vi "autobroadsidev4.vi"() -> ()   [LabVIEW 2012, in "MainProject.lvrbt"]
uses:
  MainProject.lvrbt
  <vilib>/NXT/Dual Mode Library/Waits/Wait_Num(msec).vi
  <vilib>/NXT/Hardware/Plugins/Tetrix DC Motor/TetrixDCMotorAddress.ctl
  <vilib>/NXT/LegoClasses/BrickReference/BrickReference.lvclass
  <vilib>/NXT/Subs/LVHSConnector.ctl
  <vilib>/NXT/NXTIO Xnodes/NXTIONodeSubVIs/TETRIX IO Check Battery.vi
  <vilib>/NXT/NXTIO Xnodes/NXTIOXNode/NXTIO.xnode
  <vilib>/NXT/NXTIO Xnodes/AddressXNode/NXTIOAddress.xnode
  <vilib>/NXT/NXTIO Xnodes/NXTIONodeSubVIs/TETRIX IO Stop DC Motors.vi
  Drivers/AutoControl3.ctl
  <vilib>/NXT/Block Support/NXT_InputPort.ctl
  <vilib>/NXT/HiTechnic/HiTechnic Controls/HiTechnic Port.ctl
  Drivers/AutoDriverControl.ctl
  FTC 2012 - 2013/Controls/SpeedControl.ctl
  <vilib>/NXT/Dual Mode Library/Sound/Tone.vi
  <vilib>/NXT/Dual Mode Library/Waits/Wait_Num.vi
  <vilib>/NXT/Hardware/Plugins/Tetrix 180 deg Servo/Tetrix180ServoAddress.ctl
  <vilib>/NXT/NXTIO Xnodes/NXTIONodeSubVIs/TETRIX IO Move Servos.vi
  Drivers/LineCountColorCtl.ctl
panel:
  out "Line Color":string="Black"
  in  "Dramatic Mode":bool
  out "Color":string="Black"
  out "Sector (0-9)":i16
  out "Enabled":bool
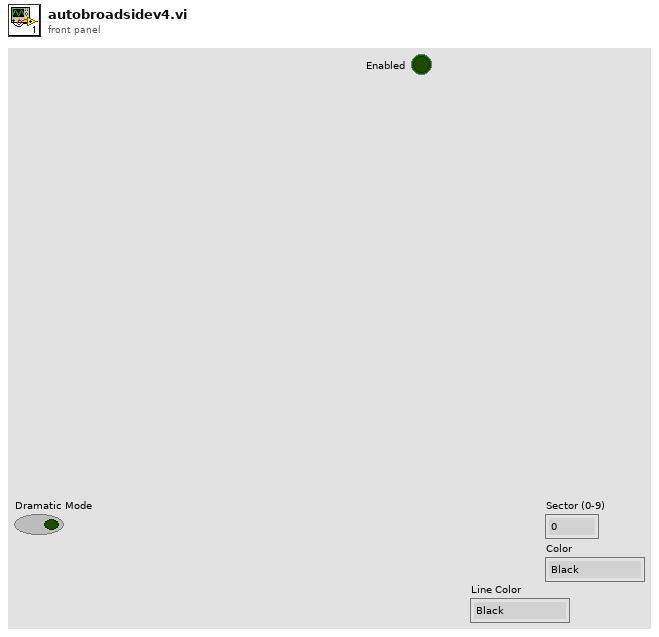
[diagram p1: front panel]
types:
  T1 = typedef "HiTechnic Port.ctl" = cluster{"Port":T2, "MUX Port":u8}
  T2 = typedef "NXT_InputPort.ctl" = u8
  T3 = typedef "TetrixDCMotorAddress.ctl" = i16
  T4 = typedef "LVHSConnector.ctl" = refnum<class "BrickReference.lvclass">
  T5 = typedef "Tetrix180ServoAddress.ctl" = i16
  T6 = typedef "AutoDriverControl.ctl" = enum16{"Init", "Forward", "Reverse", "Left", "Right", "Brake"}
  T7 = typedef "AutoControl3.ctl" = enum16{"FindIRBasket", "DropBLK", "DrvToEndOfBaskets", "DrvAroundBaskets", "AlignWithRamp", "ParkOnRamp", "Stop"}
  T8 = cluster{"Tetrix180Servo":T5, "Tetrix180Servo 2":T5, "Tetrix180Servo 3":T5, "Tetrix180Servo 4":T5}
  T9 = typedef "LineCountColorCtl.ctl" = enum16{"Init/Reset", "Check"}
  T10 = typedef "SpeedControl.ctl" = enum16{"Fast", "Medium", "Slow"}
  T11 = cluster{"Tetrix180Servo":T5, "Tetrix180Servo":T5, "Tetrix180Servo":T5, "Tetrix180Servo":T5}
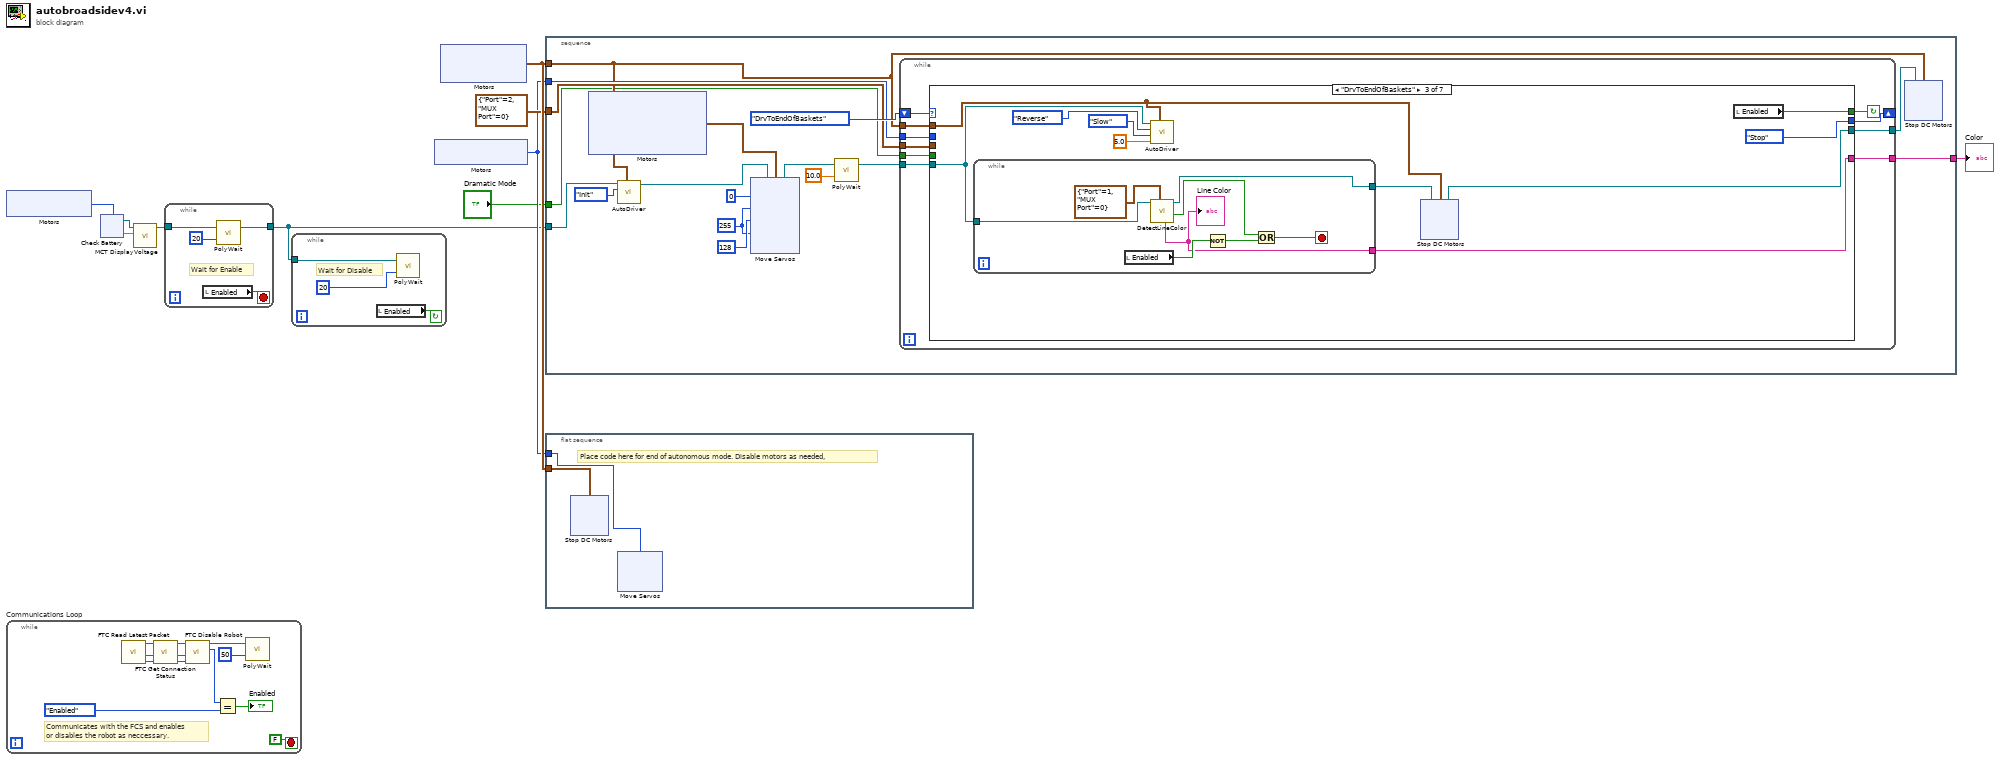
[diagram p0: block diagram]
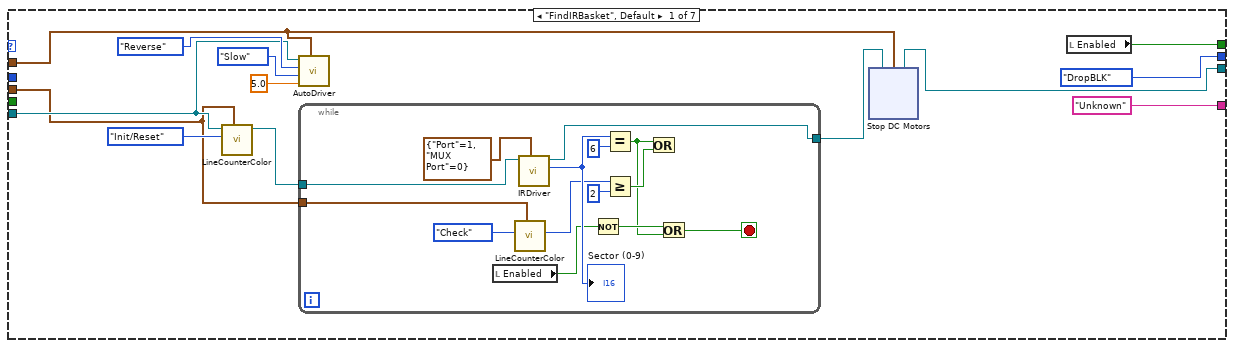
[diagram p2: hidden frame]
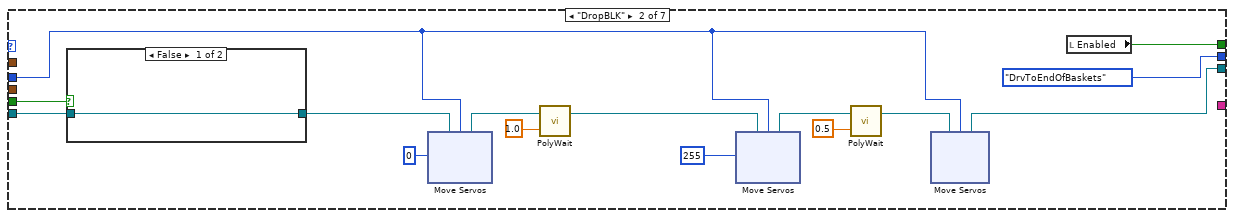
[diagram p3: hidden frame]
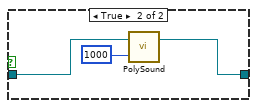
[diagram p4: hidden frame]
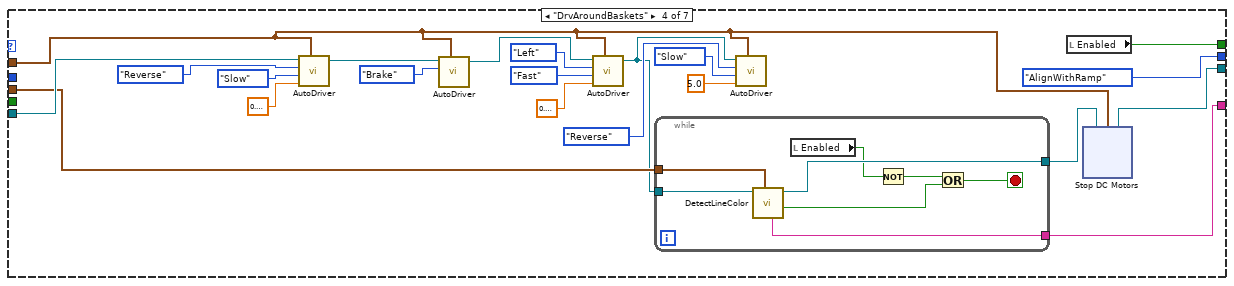
[diagram p5: hidden frame]
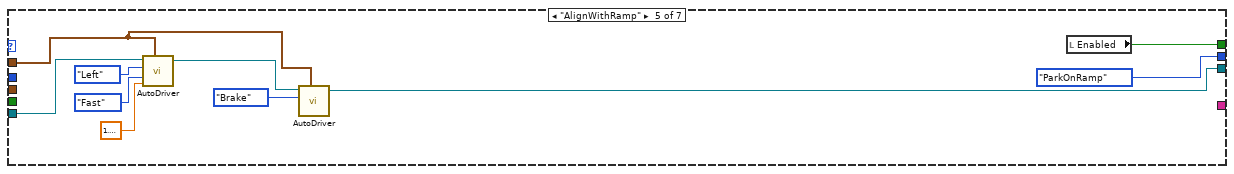
[diagram p6: hidden frame]
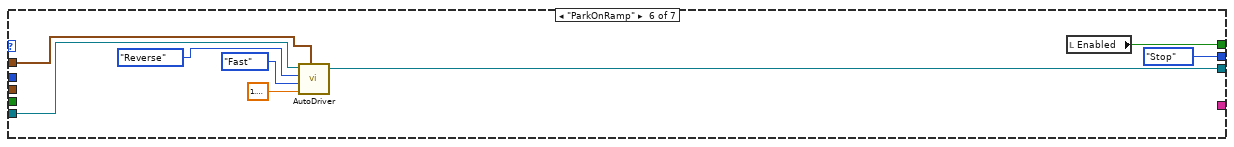
[diagram p7: hidden frame]
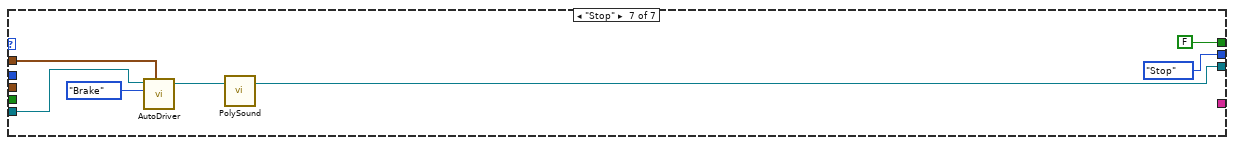
[diagram p8: hidden frame]
diagram:
  n1 = xnode "Motors"() -> ("Motor"=w5:T3)
  n2 = while "Communications Loop" {
    stop <- FALSE stop-if-true
    # "Communicates with the FCS and enables \nor disables the robot as neccessary."
    n3 = call <vilib>:"FTC Read Latest Packet.vi"() -> ("Packet Received?"=w20:bool, "Stopped?"=w19:bool, "NXT"=w22:T4)  [unwired: 6 in, 3 out]
    n4 = call <vilib>:"FTC Get Connection Status.vi"("Packet Received?"=w20, "Stopped?"=w19, "NXT"=w22) -> ("Online?"=w12:bool, "Stopped?"=w13:bool, "NXT"=w21:T4)  [unwired: 5 in]
    n5 = call <vilib>:"FTC Disable Robot.vi"("Online?"=w12, "Stopped?"=w13, "NXT"=w21) -> ("Enabled?"=w15:enum16{"Disabled", "Enabled"}, "NXT"=w17:T4)  [unwired: 3 in]
    n6 = Equal?(x=w15, y=enum16{"Disabled", "Enabled"}."Enabled") -> (x = y?=→"Enabled":bool)
    n7 = call-poly <vilib>:"PolyWait.vi"("Time (100 msec)"=u32 50 ("Time (msec)"), "NXT"=w17) -> ()  [unwired: 2 in, 1 out]
  }
  n8 = xnode "Check Battery"("Motors"=w5) -> ("Voltage 1"=w9:sgl, "NXT"=w10:T4)  [unwired: 1 in]
  n9 = call <vilib>:"MCT DisplayVoltage.vi"("Motor Voltage"=w9, "NXT"=w10) -> ("NXT"=w8:T4)  [unwired: 9 in]
  n10 = while {
    tunnel: [w25] -> w2
    tunnel: w8 -> [w23]
    stop <- w24 stop-if-true
    # "Wait for Enable"
    n11 = local read "Enabled"() -> (w24:bool)
    n12 = call-poly <vilib>:"PolyWait.vi"("Time (100 msec)"=u32 20 ("Time (msec)"), "NXT"=w23) -> ("NXT"=w25:T4)  [unwired: 2 in]
  }
  n13 = while {
    tunnel: w2 -> [w27]
    stop <- w29 continue-if-true
    # "Wait for Disable"
    n14 = local read "Enabled"() -> (w29:bool)
    n15 = call-poly <vilib>:"PolyWait.vi"("Time (100 msec)"=u32 20 ("Time (msec)"), "NXT"=w27) -> ()  [unwired: 2 in, 1 out]
  }
  n16 = xnode "Motors"() -> ("Motor"=w4:T5)
  n17 = xnode "Motors"() -> ("Motor"=w7:cluster{"TetrixDCMotor":T3, "TetrixDCMotor":T3})
  n18 = stacked-sequence {
    tunnel: w7 -> [w39]
    tunnel: w2 -> [w44]
    tunnel: T1 {"Port"=2, "MUX Port"=0} ("Port/MUX") -> [w45]
    tunnel: w4 -> [w41]
    tunnel: [w40] -> w3
    tunnel: "Dramatic Mode" -> [w30]
    frame #0 {
      w33 = u8 255 ("Position 2")
      n19 = xnode "Motors"() -> ("Motor"=w36:T11)
      n20 = call "AutoDriver.vi"("NXT In"=w44, "Motors"=w39, "Direction"=AutoDriverControl."Init") -> ("NXT Out"=w43:T4)  [unwired: 5 in]
      n21 = xnode "Move Servos"("Position 4"=w33, "Position 3"=u8 128 ("Position 5"), "Position 2"=w33, "Position 1"=u8 0, "Servos"=w36, "NXT"=w43) -> ("NXT"=w37:T4)
      n22 = call-poly <vilib>:"PolyWait.vi"("Time (1 sec)"=sgl 10.0, "NXT"=w37) -> ("NXT"=w32:T4)  [unwired: 2 in]
      n23 = while {
        tunnel: w39 -> [w78]
        tunnel: w32 -> [w77]
        shift-right: [w76] -> _
        shift-left: AutoControl3."DrvToEndOfBaskets" -> [w75]
        tunnel: w45 -> [w74]
        tunnel: w41 -> [w72]
        tunnel: [w71] -> w40
        tunnel: [w70] -> w38
        tunnel: w30 -> [w69]
        stop <- w73 continue-if-true
        n24 = case shown="\"DrvToEndOfBaskets\"" w75 {
          tunnel: w78 -> [w86 _ w154 w178 w215 w230 w238]
          tunnel: w77 -> [w87 w120 w155 w198 w214 w231 w237]
          tunnel: [AutoControl3."DropBLK" AutoControl3."DrvToEndOfBaskets" AutoControl3."Stop" AutoControl3."AlignWithRamp" AutoControl3."ParkOnRamp" AutoControl3."Stop" AutoControl3."Stop"] -> w76
          tunnel: w74 -> [w79 _ _ w191 _ _ _]
          tunnel: [w83 w119 w161 w185 w217 w225 FALSE] -> w73
          tunnel: w72 -> [_ w114 _ _ _ _ _]
          tunnel: ["Unknown" ("Color") _ w153 w186 _ _ _] -> w71
          tunnel: [w82 w118 w156 w179 w216 w224 w232] -> w70
          tunnel: w69 -> [_ w113 _ _ _ _ _]
          frame "FindIRBasket", Default {
            n25 = call "LineCounterColor.vi"("Port/MUX"=w79, "Enum"=LineCountColorCtl."Init/Reset", "NXT In"=w87) -> ("NXT Out"=w81:T4)  [unwired: 7 in, 1 out]
            n26 = call "AutoDriver.vi"("NXT In"=w87, "Motors"=w86, "Direction"=AutoDriverControl."Reverse", "Speed"=SpeedControl."Slow", "Time (1 sec)"=sgl 5.0) -> ()  [unwired: 3 in, 1 out]
            n27 = while {
              tunnel: w81 -> [w109]
              tunnel: w79 -> [w105]
              tunnel: [w106] -> w84
              stop <- w102 stop-if-true
              n28 = local read "Enabled"() -> (w103:bool)
              n29 = call "LineCounterColor.vi"("Port/MUX"=w105, "Enum"=LineCountColorCtl."Check") -> ("Numeric"=w100:i16)  [unwired: 8 in, 1 out]
              n30 = call "IRDriver.vi"("Port"=T1 {"Port"=1, "MUX Port"=0}, "NXT In"=w109) -> ("Sector (0-9)"=w111:i16, "NXT Out"=w106:T4)  [unwired: 8 in]
              "Sector (0-9)" <- w111
              n31 = Not(x=w103) -> (.not. x?=w101:bool)
              n32 = Equal?(x=w111, y=i16 6) -> (x = y?=w99:bool)
              n33 = Greater Or Equal?(x=w100, y=i16 2) -> (x >= y?=w107:bool)
              n34 = Or(x=w99, y=w107) -> ()  [unwired: 1 out]
              n35 = Or(x=w101, y=w99) -> (x .or. y?=w102:bool)
            }
            n36 = xnode "Stop DC Motors"("Motors"=w86, "NXT"=w84) -> ("NXT"=w82:T4)
            n37 = local read "Enabled"() -> (w83:bool)
          }
          frame "DropBLK" {
            n38 = case shown="False" w113 {
              tunnel: w120 -> [w128 w130]
              tunnel: [w128 w129] -> w116
              frame False {
              }
              frame True {
                n39 = call-poly <vilib>:"PolySound.vi"("Duration (500 ms)"=u16 1000, "NXT"=w130) -> ("NXT"=w129:T4)  [unwired: 2 in]
              }
            }
            n40 = xnode "Move Servos"("Position 1"=u8 0, "Servos"=w114, "NXT"=w116) -> ("NXT"=w115:T4)
            n41 = call-poly <vilib>:"PolyWait.vi"("Time (1 sec)"=sgl 1.0, "NXT"=w115) -> ("NXT"=w125:T4)  [unwired: 2 in]
            n42 = xnode "Move Servos"("Position 1"=u8 255, "Servos"=w114, "NXT"=w125) -> ("NXT"=w124:T4)
            n43 = call-poly <vilib>:"PolyWait.vi"("Time (1 sec)"=sgl 0.5, "NXT"=w124) -> ("NXT"=w121:T4)  [unwired: 2 in]
            n44 = xnode "Move Servos"("Servos"=w114, "NXT"=w121) -> ("NXT"=w118:T4)  [unwired: 1 in]
            n45 = local read "Enabled"() -> (w119:bool)
          }
          frame "DrvToEndOfBaskets" {
            n46 = while {
              tunnel: w155 -> [w176]
              tunnel: [w175] -> w157
              tunnel: [w170] -> w153
              stop <- w173 stop-if-true
              n47 = local read "Enabled"() -> (w174:bool)
              n48 = call "DetectLineColor.vi"("Port/MUX"=T1 {"Port"=1, "MUX Port"=0} ("Port"), "NXT In"=w176) -> ("Detected Line?"=w171:bool, "NXT Out"=w175:T4, "Color"=w170:string)  [unwired: 7 in]
              "Line Color" <- w170
              n49 = Not(x=w174) -> (.not. x?=w172:bool)
              n50 = Or(x=w171, y=w172) -> (x .or. y?=w173:bool)
            }
            n51 = call "AutoDriver.vi"("NXT In"=w155, "Motors"=w154, "Direction"=AutoDriverControl."Reverse", "Speed"=SpeedControl."Slow", "Time (1 sec)"=sgl 5.0) -> ()  [unwired: 3 in, 1 out]
            n52 = xnode "Stop DC Motors"("Motors"=w154, "NXT"=w157) -> ("NXT"=w156:T4)
            n53 = local read "Enabled"() -> (w161:bool)
          }
          frame "DrvAroundBaskets" {
            n54 = call "AutoDriver.vi"("NXT In"=w198, "Motors"=w178, "Direction"=AutoDriverControl."Reverse", "Speed"=SpeedControl."Slow", "Time (1 sec)"=sgl 0.3) -> ("NXT Out"=w189:T4)  [unwired: 3 in]
            n55 = call "AutoDriver.vi"("NXT In"=w189, "Motors"=w178, "Direction"=AutoDriverControl."Brake") -> ("NXT Out"=w188:T4)  [unwired: 5 in]
            n56 = call "AutoDriver.vi"("NXT In"=w188, "Motors"=w178, "Direction"=AutoDriverControl."Left", "Speed"=SpeedControl."Fast", "Time (1 sec)"=sgl 0.8) -> ("NXT Out"=w181:T4)  [unwired: 3 in]
            n57 = while {
              tunnel: w191 -> [w213]
              tunnel: [w212] -> w186
              tunnel: [w211] -> w180
              tunnel: w181 -> [w206]
              stop <- w208 stop-if-true
              n58 = call "DetectLineColor.vi"("Port/MUX"=w213, "NXT In"=w206) -> ("Detected Line?"=w209:bool, "NXT Out"=w211:T4, "Color"=w212:string)  [unwired: 7 in]
              n59 = local read "Enabled"() -> (w210:bool)
              n60 = Not(x=w210) -> (.not. x?=w207:bool)
              n61 = Or(x=w207, y=w209) -> (x .or. y?=w208:bool)
            }
            n62 = call "AutoDriver.vi"("NXT In"=w181, "Motors"=w178, "Direction"=AutoDriverControl."Reverse", "Speed"=SpeedControl."Slow", "Time (1 sec)"=sgl 5.0) -> ()  [unwired: 3 in, 1 out]
            n63 = local read "Enabled"() -> (w185:bool)
            n64 = xnode "Stop DC Motors"("Motors"=w178, "NXT"=w180) -> ("NXT"=w179:T4)
          }
          frame "AlignWithRamp" {
            n65 = call "AutoDriver.vi"("NXT In"=w214, "Motors"=w215, "Direction"=AutoDriverControl."Left", "Speed"=SpeedControl."Fast", "Time (1 sec)"=sgl 1.1) -> ("NXT Out"=w219:T4)  [unwired: 3 in]
            n66 = call "AutoDriver.vi"("NXT In"=w219, "Motors"=w215, "Direction"=AutoDriverControl."Brake") -> ("NXT Out"=w216:T4)  [unwired: 5 in]
            n67 = local read "Enabled"() -> (w217:bool)
          }
          frame "ParkOnRamp" {
            n68 = call "AutoDriver.vi"("NXT In"=w231, "Motors"=w230, "Direction"=AutoDriverControl."Reverse", "Speed"=SpeedControl."Fast", "Time (1 sec)"=sgl 1.3) -> ("NXT Out"=w224:T4)  [unwired: 3 in]
            n69 = local read "Enabled"() -> (w225:bool)
          }
          frame "Stop" {
            n70 = call "AutoDriver.vi"("NXT In"=w237, "Motors"=w238, "Direction"=AutoDriverControl."Brake") -> ("NXT Out"=w235:T4)  [unwired: 5 in]
            n71 = call-poly <vilib>:"PolySound.vi"("NXT"=w235) -> ("NXT"=w232:T4)  [unwired: 3 in]
          }
        }
      }
      n72 = xnode "Stop DC Motors"("Motors"=w39, "NXT"=w38) -> ()  [unwired: 1 out]
    }
  }
  "Color" <- w3
  n73 = flat-sequence {
    tunnel: w7 -> [w239]
    tunnel: w4 -> [w240]
    frame #0 {
      # "Place code here for end of autonomous mode. Disable motors as needed,"
      n74 = xnode "Stop DC Motors"("Motors"=w239) -> ()  [unwired: 1 in, 1 out]
      n75 = xnode "Move Servos"("Servos"=w240) -> ()  [unwired: 2 in, 1 out]
    }
  }
